vi "AdvanceIR.vi"(7 "stop":bool, 8 "error in (no error)":errorcluster, 9 "PID gains":T1={"proportional gain (Kc)"=5.0, "integral time (Ti, min)"=0.0, "derivative time (Td, min)"=0.0}, 10 "side":dbl=75.0 format="%#_13g", 11 "straight":dbl=75.0 format="%#_13g") -> (0 "error out":errorcluster, 3 "誤差":dbl)   [LabVIEW 2018]
uses:
  <vilib>/Platform/TimedLoop/XDataNode/timing_clust.ctl
  <vilib>/Platform/TimedLoop/XDataNode/nitl_modes.ctl
  <vilib>/Platform/TimedLoop/XDataNode/wakeup.ctl
  <vilib>/addons/control/pid/pid.llb/PID (DBL).vi
  <vilib>/platform/TimedLoop/XDataNode/XDataNode.xnode
  <vilib>/Platform/TimedLoop/XDataNode/XDNodeRunTimeDep.lvlib
  <vilib>/addons/control/pid/NI_PID_pid.lvlib
panel:
  out "絕對誤差":dbl
  in  "second":i32
  out "times":i32
  out "IR":dbl[](array[numeric])
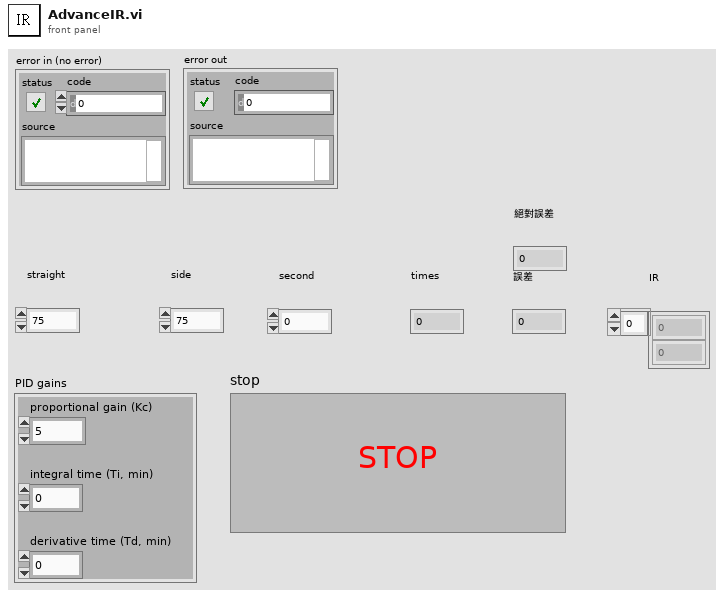
[diagram p1: front panel]
types:
  T1 = cluster{"proportional gain (Kc)":dbl, "integral time (Ti, min)":dbl, "derivative time (Td, min)":dbl}
  T2 = typedef "XDNodeRunTimeDep.lvlib/timing_clust.ctl" = cluster{"Expected End [f-1]":u64, "Actual End [f-1]":u64, "Finished Late? [f-1]":bool, "Expected End [i-1]":u64, "Actual End [i-1]":u64, "Finished Late? [i-1]":bool, "Expected Start [i]":u64, "Actual Start [i]":u64, "Expected Start [f]":u64, "Actual Start [f]":u64, "Source Name":string, "Structure Name":string, "Period":i64, "Deadline":i64, "Offset":i64, "Start":i64, "Priority":i32, "Timeout":i32, "Mode":T3, "Wakeup Reason":T4, "Error":errorcluster, "Source Type":string, "Secondary Source Type":string, "Global End Time":u64, "Global Start Time":u64, "Frame Duration":u64, "Iteration Duration":u64, "Assigned CPU":i32, "I/O Scan Engine Mode":u32}
  T3 = typedef "XDNodeRunTimeDep.lvlib/nitl_modes.ctl" = enum32{"No Change", "Process missed periods, maintain original phase", "Discard missed periods, maintain original phase", "Process missed periods, ignore original phase", "Discard missed periods, ignore original phase"}
  T4 = typedef "XDNodeRunTimeDep.lvlib/wakeup.ctl" = enum32{"Normal", "Aborted", "Asynchronous wakeup", "Timing source error", "Timed loop error", "Timeout"}
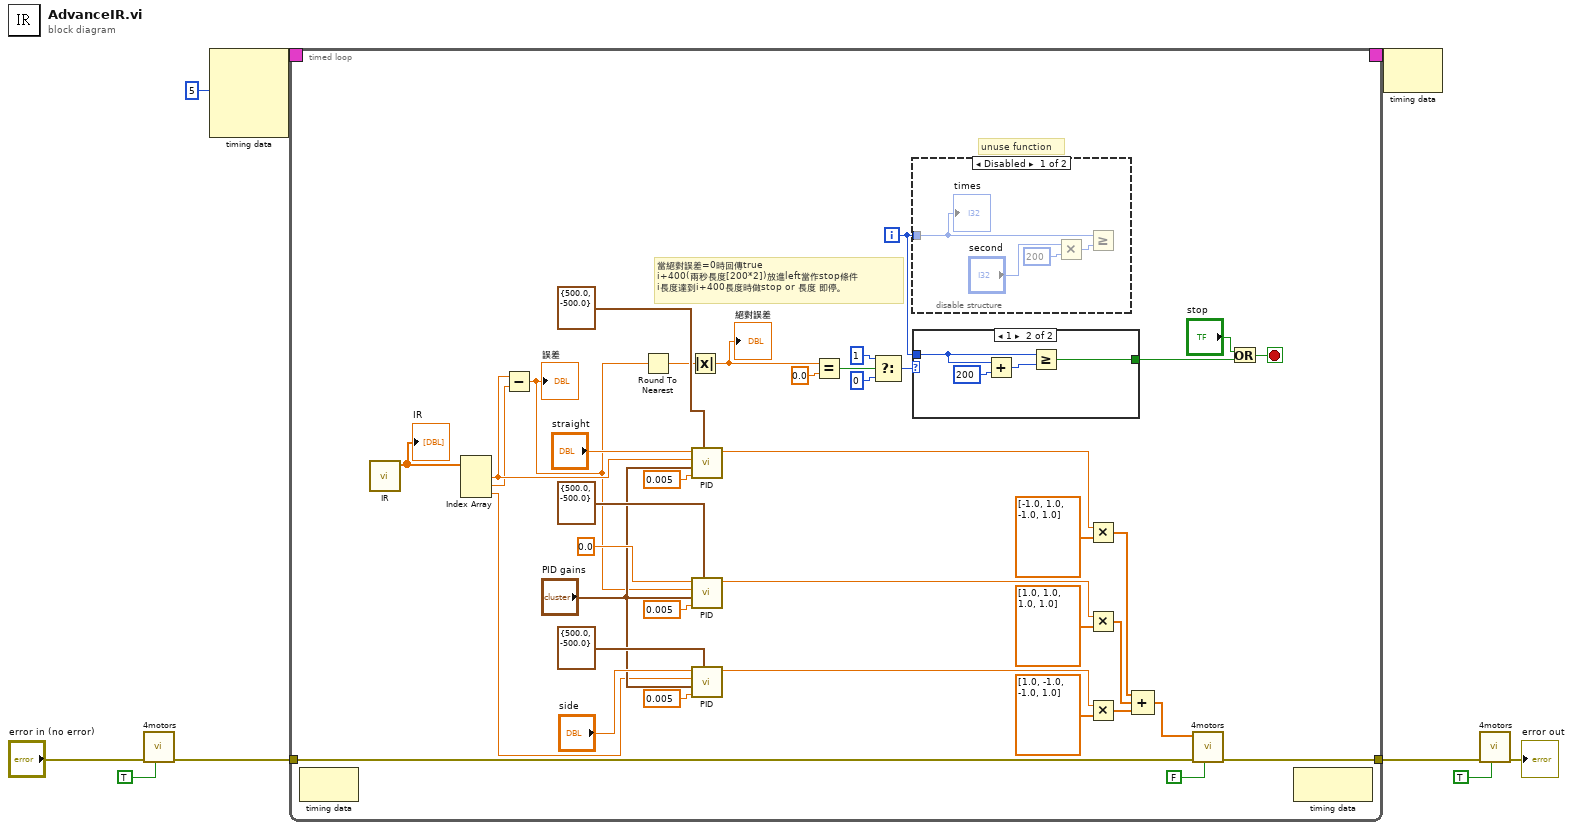
[diagram p0: block diagram]
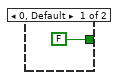
[diagram p2: hidden frame]
diagram:
  n1 = call "4motors.vi"("Reset"=TRUE, "error in (no error)"="error in (no error)") -> ("error out"=w5:errorcluster)  [unwired: 8 in, 1 out]
  n2 = node-c288(i64 5 ("Period")) -> (w9:T2)  [unwired: 3 in]
  n3 = timed-loop {
    timing: w9 -> [_]
    timing-out: [_] -> w8
    tunnel: [w44] -> w6
    tunnel: w5 -> [w14]
    i -> [w11]
    stop <- w13 stop-if-true
    # "unuse function"
    # "當絕對誤差=0時回傳true\ni+400(兩秒長度[200*2])放進left當作stop條件\ni長度達到i+400長度時做stop or 長度 即停。"
    n4 = node-c288() -> ()  [unwired: 1 in, 1 out]
    n5 = call "IR.vi"() -> ("IR"=w48:dbl[])  [unwired: 10 in, 1 out]
    "IR" <- w48
    n6 = Index Array(array=w48) -> (element #1=w42:dbl, element #2=w41:dbl, element #3=w25:dbl)  [unwired: 3 in]
    n7 = Subtract(x=w42, y=w41) -> (x-y=w21:dbl)
    "誤差" <- w21
    n8 = Round To Nearest(number=w21) -> (nearest integer value=w20:dbl)
    n9 = Absolute Value(x=w20) -> (abs(x)=w16:dbl)
    "絕對誤差" <- w16
    n10 = call-poly <vilib>:"PID.vi"("output range"=cluster{"output high":dbl, "output low":dbl} {"output high"=500.0, "output low"=-500.0}, "dt (s)"=0.005, "PID gains"="PID gains", "process variable"=w42, "setpoint"="straight") -> ("output"=w45:dbl)  [unwired: 5 in, 1 out]
    n11 = call-poly <vilib>:"PID.vi"("output range"=cluster{"output high":dbl, "output low":dbl} {"output high"=500.0, "output low"=-500.0}, "dt (s)"=0.005, "PID gains"="PID gains", "process variable"=w21, "setpoint"=0.0) -> ("output"=w34:dbl)  [unwired: 5 in, 1 out]
    n12 = call-poly <vilib>:"PID.vi"("output range"=cluster{"output high":dbl, "output low":dbl} {"output high"=500.0, "output low"=-500.0}, "dt (s)"=0.005, "PID gains"="PID gains", "process variable"=w25, "setpoint"="side") -> ("output"=w37:dbl)  [unwired: 5 in, 1 out]
    n13 = Equal?(x=w16, y=0.0) -> (x = y?=w17:bool)
    n14 = Select(t=1, s=w17, f=0) -> (s? t:f=w12:i32)
    n15 = disable-structure shown="Disabled" {
      disable-tunnel: w11 -> [w57 _]
      frame Disabled {
        n16 = Multiply(x="second", y=200) -> (x*y=w54:i32)
        n17 = Greater Or Equal?(x=w57, y=w54) -> ()  [unwired: 1 out]
        "times" <- w57
      }
      frame Enabled {
      }
    }
    n18 = case shown="1" w12 {
      tunnel: w11 -> [_ w51]
      tunnel: [FALSE w50] -> w10
      frame 0, Default {
      }
      frame 1 {
        n19 = Add(x=w51, y=200) -> (x+y=w52:i32)
        n20 = Greater Or Equal?(x=w51, y=w52) -> (x >= y?=w50:bool)
      }
    }
    n21 = Multiply(x=w45, y=dbl[] [-1.0, 1.0, -1.0, 1.0] ("IR")) -> (x*y=w28:dbl[])
    n22 = Multiply(x=w34, y=dbl[] [1.0, 1.0, 1.0, 1.0] ("IR")) -> (x*y=w29:dbl[])
    n23 = Multiply(x=w37, y=dbl[] [1.0, -1.0, -1.0, 1.0] ("IR")) -> (x*y=w30:dbl[])
    n24 = Compound Arithmetic op=ADD(w28, w29, w30) -> (w27:dbl[])
    n25 = call "4motors.vi"("Reset"=FALSE, "error in (no error)"=w14, "Power"=w27) -> ("error out"=w44:errorcluster)  [unwired: 7 in, 1 out]
    n26 = Or(x="stop", y=w10) -> (x .or. y?=w13:bool)
    n27 = node-c288() -> ()  [unwired: 1 in, 1 out]
  }
  n28 = node-c288(w8) -> ()  [unwired: 1 out]
  n29 = call "4motors.vi"("Reset"=TRUE, "error in (no error)"=w6) -> ("error out"=→"error out":errorcluster)  [unwired: 8 in, 1 out]
